vi "Performance test.vi"() -> ()   [LabVIEW 2017]
panel:
  out "x-y":u32
  # "100 calls with 1000 strings"
  # "Both changed 7400 ms"
  # "Deleted more indicators and 5500ms"
  # "Extensive use of Inplace Struct 2160ms"
  # "Use Variant imple 430ms"
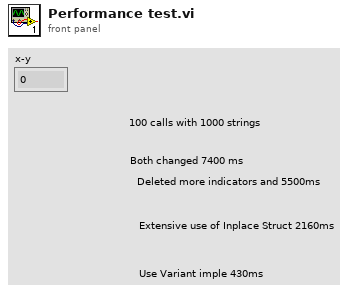
[diagram p1: front panel]
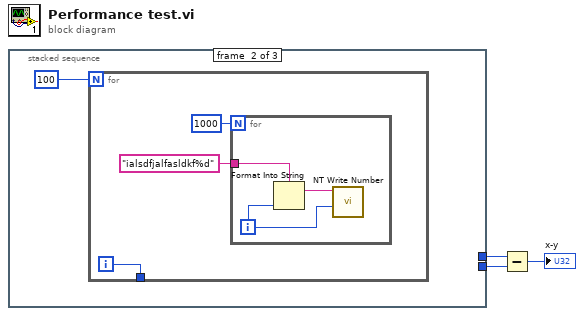
[diagram p0: block diagram]
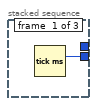
[diagram p2: hidden frame]
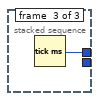
[diagram p3: hidden frame]
diagram:
  n1 = stacked-sequence {
    tunnel: [w4 _ _] -> w3
    tunnel: [_ _ w12] -> w2
    frame #0 {
      n2 = Tick Count (ms)() -> (millisecond timer value=w4:u32)
    }
    frame #1 {
      n3 = for {
        N: 100 -> [_]
        tunnel: [w6] -> _
        i -> [w6]
        n4 = for {
          N: 1000 -> [_]
          tunnel: "ialsdfjalfasldkf%d" ("Field") -> [w11]
          i -> [w10]
          n5 = Format Into String(format string=w11, w10) -> (resulting string=w9:string)  [unwired: 2 in, 1 out]
          n6 = call <vilib>:"NT Write Number.vi"("Numeric"=w10, "Name"=w9) -> ()  [unwired: 9 in, 1 out]
        }
      }
    }
    frame #2 {
      n7 = Tick Count (ms)() -> (millisecond timer value=w12:u32)
    }
  }
  n8 = Subtract(x=w2, y=w3) -> (x-y=→"x-y":u32)
